vi "Vibrate Joystick Based on Match Time.vi"(1 "error in":errorcluster) -> (0 "Remanining Match Time(s)":sgl)   [LabVIEW 2015]
uses:
  <vilib>/Rock Robotics/WPI/Utilities/WPI_GetSetVariantRefNum.vi
  <vilib>/Rock Robotics/WPI/Joystick/WPI_JoystickDeviceEnum.ctl
panel:
  in  "Remaining Match Time":dbl format="%#_13g"
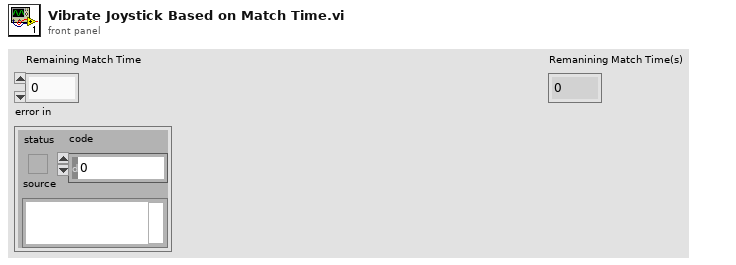
[diagram p1: front panel]
types:
  T1 = typedef "WPI_JoystickDevRef.ctl" = cluster{"Device":T2}
  T2 = typedef "WPI_JoystickDeviceEnum.ctl" = enum16{"USB 0", "USB 1", "USB 2", "USB 3", "USB 4", "USB 5"}
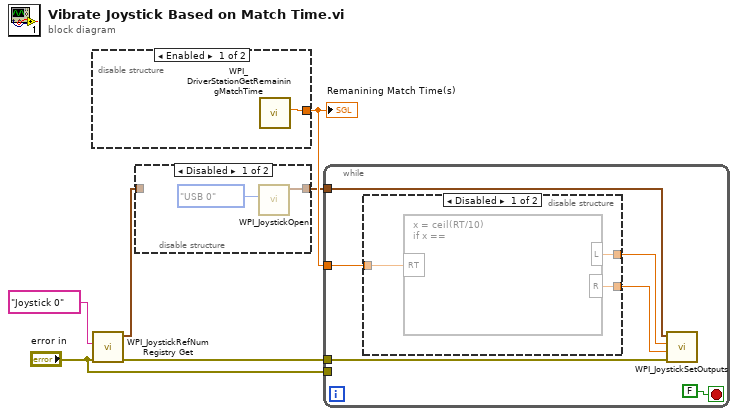
[diagram p0: block diagram]
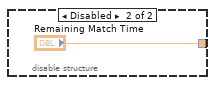
[diagram p3: hidden frame]
diagram:
  n1 = disable-structure shown="Enabled" {
    disable-tunnel: [w7 "Remaining Match Time"] -> w4
    frame Enabled {
      n2 = call <vilib>:"WPI_DriverStationGetRemainingMatchTime.vi"() -> ("Match Time(s)"=w7:sgl)  [unwired: 10 in, 1 out]
    }
    frame Disabled {
    }
  }
  "Remanining Match Time(s)" <- w4
  n3 = call <vilib>:"WPI_JoystickRefNum Registry Get.vi"("error in (no error)"="error in", "refnum name"="Joystick 0") -> ("error out"=w5:errorcluster, "JoystickDevRef"=w2:T1)  [unwired: 8 in]
  n4 = disable-structure shown="Disabled" {
    disable-tunnel: [w9 w11] -> w3
    disable-tunnel: w2 -> [_ w11]
    frame Disabled {
      n5 = call <vilib>:"WPI_JoystickOpen.vi"("JoystickDevice"=WPI_JoystickDeviceEnum."USB 0") -> ("JoystickDevRef"=w9:T1)  [unwired: 10 in]
    }
    frame Enabled {
    }
  }
  n6 = while {
    tunnel: w3 -> [w17]
    tunnel: w5 -> [w16]
    tunnel: w4 -> [w14]
    tunnel: "error in" -> [_]
    stop <- FALSE stop-if-true
    n7 = disable-structure shown="Disabled" {
      disable-tunnel: w14 -> [w20 _]
      disable-tunnel: [w19 _] -> w13
      disable-tunnel: [w18 _] -> w12
      frame Disabled {
        n8 = formula code="x = ceil(RT/10)\nif x =="("RT"=w20) -> ("L"=w19:dbl, "R"=w18:dbl)
      }
      frame Enabled {
      }
    }
    n9 = call <vilib>:"WPI_JoystickSetOutputs.vi"("error in (no error)"=w16, "Right Rumble"=w12, "Left Rumble"=w13, "JoystickDevRef"=w17) -> ()  [unwired: 6 in, 2 out]
  }
